vi "OutputShooter.vi"() -> ()   [LabVIEW 2023]
doc: "This VI sends commands to the arm subsystem."
uses:
  f035948c-00ce-4b24-a9d1-78143a22adfc.vi
  GlobalShooter.vi
  GRNF_CTREMotor.vi
  <vilib>/Rock Robotics/WPI/ThirdParty/Phoenix-LabVIEW/Motor Controller/Get/CTRE_Phoenix_MotorController_GetSelectedSensorData.vi
  <vilib>/Rock Robotics/WPI/ThirdParty/Phoenix-LabVIEW/Motor Controller/Get/CTRE_Phoenix_MotorController_GetVoltage.vi
  <vilib>/Rock Robotics/Network Tables/NT Read Number.vi
  <vilib>/Rock Robotics/Network Tables/NT Read Boolean.vi
  <vilib>/Rock Robotics/WPI/ThirdParty/Phoenix-LabVIEW/Motor Controller/Get/CTRE_Phoenix_MotorController_GetGeneralStatus.vi
  GlobalDriverStationData.vi
  GlobalElevator.vi
  GlobalDriverStationCommands.vi
panel:
  in  "Wrist Homing Power":dbl=-0.1 format="%#_13g"
  in  "Shootering?":bool=TRUE
  in  "OUT_Wrist_PID_Mode Override":T1(ring)=enum."Positioning"
  out "Error Chart":dbl(graph)=-0.3784677933673469
  out "Angle Chart":dbl(graph)=-0.3784677933673469
  out "Wrist Error":dbl=-0.3784677933673469
  in  "Wrist output override":bool
  in  "OUT_Shooter_Wrist":dbl
  in  "Shooter Right PID Configuration":T2
  in  "Shooter Left PID Configuration":T2
  in  "Manual Shooter Right Speed Goal (rpm)":dbl min=0.0 max=6000.0 step=100.0
  in  "Manual Shooter Left Speed Goal (rpm)":dbl min=0.0 max=6000.0 step=100.0
  in  "Override Shooter State Controller":bool
  out "Shooter Right":T3(graph)
  out "Shooter Left":T3(graph)
  in  "Plot Shooter":bool
  in  "Wrist Scalar":dbl=0.008
  in  "Wrist Positioning PID Parameters":T2={"Kp"=0.060000000000000005, "Ki"=0.0, "Kd"=0.0, "Kf (don't use)"=0.0, "I-Zone"=10.0} {"Kd" min=0.0; "Ki" min=0.0; "Kp" min=0.0}
  in  "Wrist Acceleration (deg/s^2)":dbl=550.0
  in  "Wrist S-Curve Strength":dbl=4.0
  in  "Wrist Cruise Velocity (deg/s)":dbl=350.0
  in  "Wrist Travelling PID Parameters":T2={"Kp"=0.05, "Ki"=1e-05, "Kd"=0.0, "Kf (don't use)"=0.0, "I-Zone"=10.0} {"Kd" min=0.0; "Ki" min=0.0; "Kp" min=0.0}
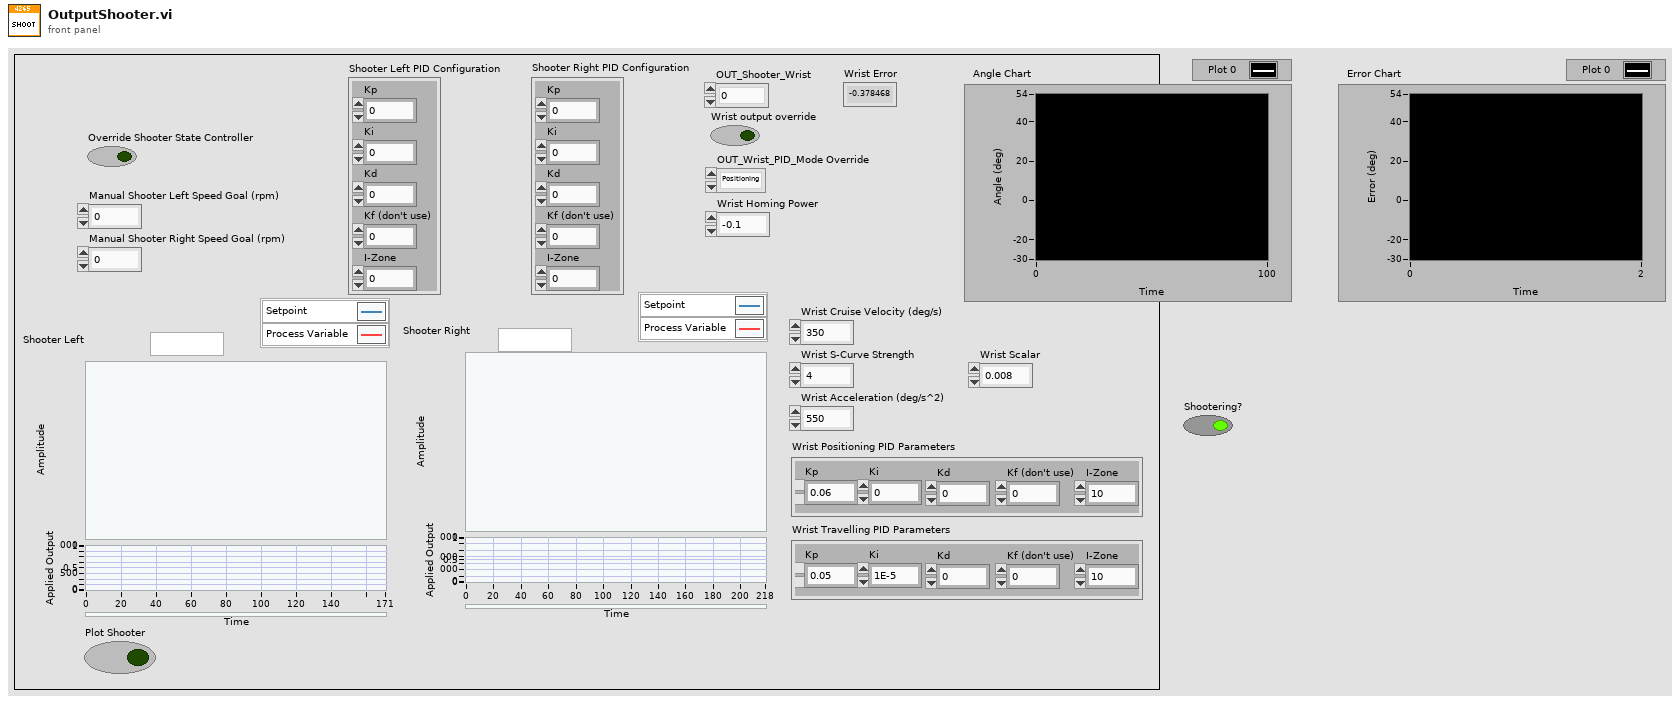
[diagram p1: front panel]
types:
  T1 = enum16{"Safety", "Travelling", "Positioning", "Holding"}
  T2 = cluster{"Kp":dbl, "Ki":dbl, "Kd":dbl, "Kf (don't use)":dbl, "I-Zone":dbl}
  T3 = cluster{"Sensor Velocity":dbl, "Setpoint":dbl, "Applied Output":dbl}
  T4 = typedef "WPI_MotorControlDeviceRef.ctl" = cluster{"DeviceStatus":errorcluster, "Type":T5, "PWM":cluster{"PWM Channel":T6, "DeadBand":T7}, "CAN":cluster{"Device Number":u8, "SetOutput VI Ref":variant, "GetOutput VI Ref":variant, "Enable VI Ref":variant, "Disable VI Ref":variant, "Data":variant}, "Invert":bool, "DIO PWM":cluster{"PWM \"Enable\" Channel":T6, "DIOChannel":T8, "PWM Rate":dbl}}
  T5 = typedef "WPI_MotorControlType.ctl" = enum16{"PWM", "CAN", "DIO PWM"}
  T6 = typedef "FPGA_DIOPWMChannel.ctl" = enum8{"PWM 0", "PWM 1", "PWM 2", "PWM 3", "PWM 4", "PWM 5", "PWM 6", "PWM 7", "PWM 8", "PWM 9", "PWM MXP 0", "PWM MXP 1", "PWM MXP 2", "PWM MXP 3", "PWM MXP 4", "PWM MXP 5", "PWM MXP 6", "PWM MXP 7", "PWM MXP 8", "PWM MXP 9", "Invalid"}
  T7 = typedef "WPI_PWMDeadband.ctl" = cluster{"Name":string, "maxPositivePwm":i32, "minPositivePwm":i32, "centerPwm":i32, "maxNegativePwm":i32, "minNegativePwm":i32, "angularRange":u16}
  T8 = typedef "FPGA_DIOChannel.ctl" = enum8{"DIO 0", "DIO 1", "DIO 2", "DIO 3", "DIO 4", "DIO 5", "DIO 6", "DIO 7", "DIO 8", "DIO 9", "DIO MXP 0", "DIO MXP 1", "DIO MXP 2", "DIO MXP 3", "DIO MXP 4", "DIO MXP 5", "DIO MXP 6", "DIO MXP 7", "DIO MXP 8", "DIO MXP 9", "DIO MXP 10", "DIO MXP 11", "DIO MXP 12", "DIO MXP 13", "DIO MXP 14", "DIO MXP 15", "SPI Port CS1", "SPI Port CS2", "SPI Port CS3", "SPI Port MISO", "SPI Port MOSI", "Invalid"}
  T9 = enum16{"No Changed Output", "New Normal Output", "New Testing Output"}
  T10 = cluster{"Interlocked Output":dbl, dbl, "Percent Output":dbl}
  T11 = typedef "WPI_SolenoidDevRef.ctl" = cluster{"DevStatus":errorcluster, "Pneumatics Control Module":u8, "Forward Solenoid Channel":T12, "Reverse Solenoid Channel":T12}
  T12 = typedef "WPI_SolenoidChannel.ctl" = enum8{"Solenoid 0", "Solenoid 1", "Solenoid 2", "Solenoid 3", "Solenoid 4", "Solenoid 5", "Solenoid 6", "Solenoid 7", "Solenoid 8", "Solenoid 9", "Solenoid 10", "Solenoid 11", "Solenoid 12", "Solenoid 13", "Solenoid 14", "Solenoid 15", "Invalid"}
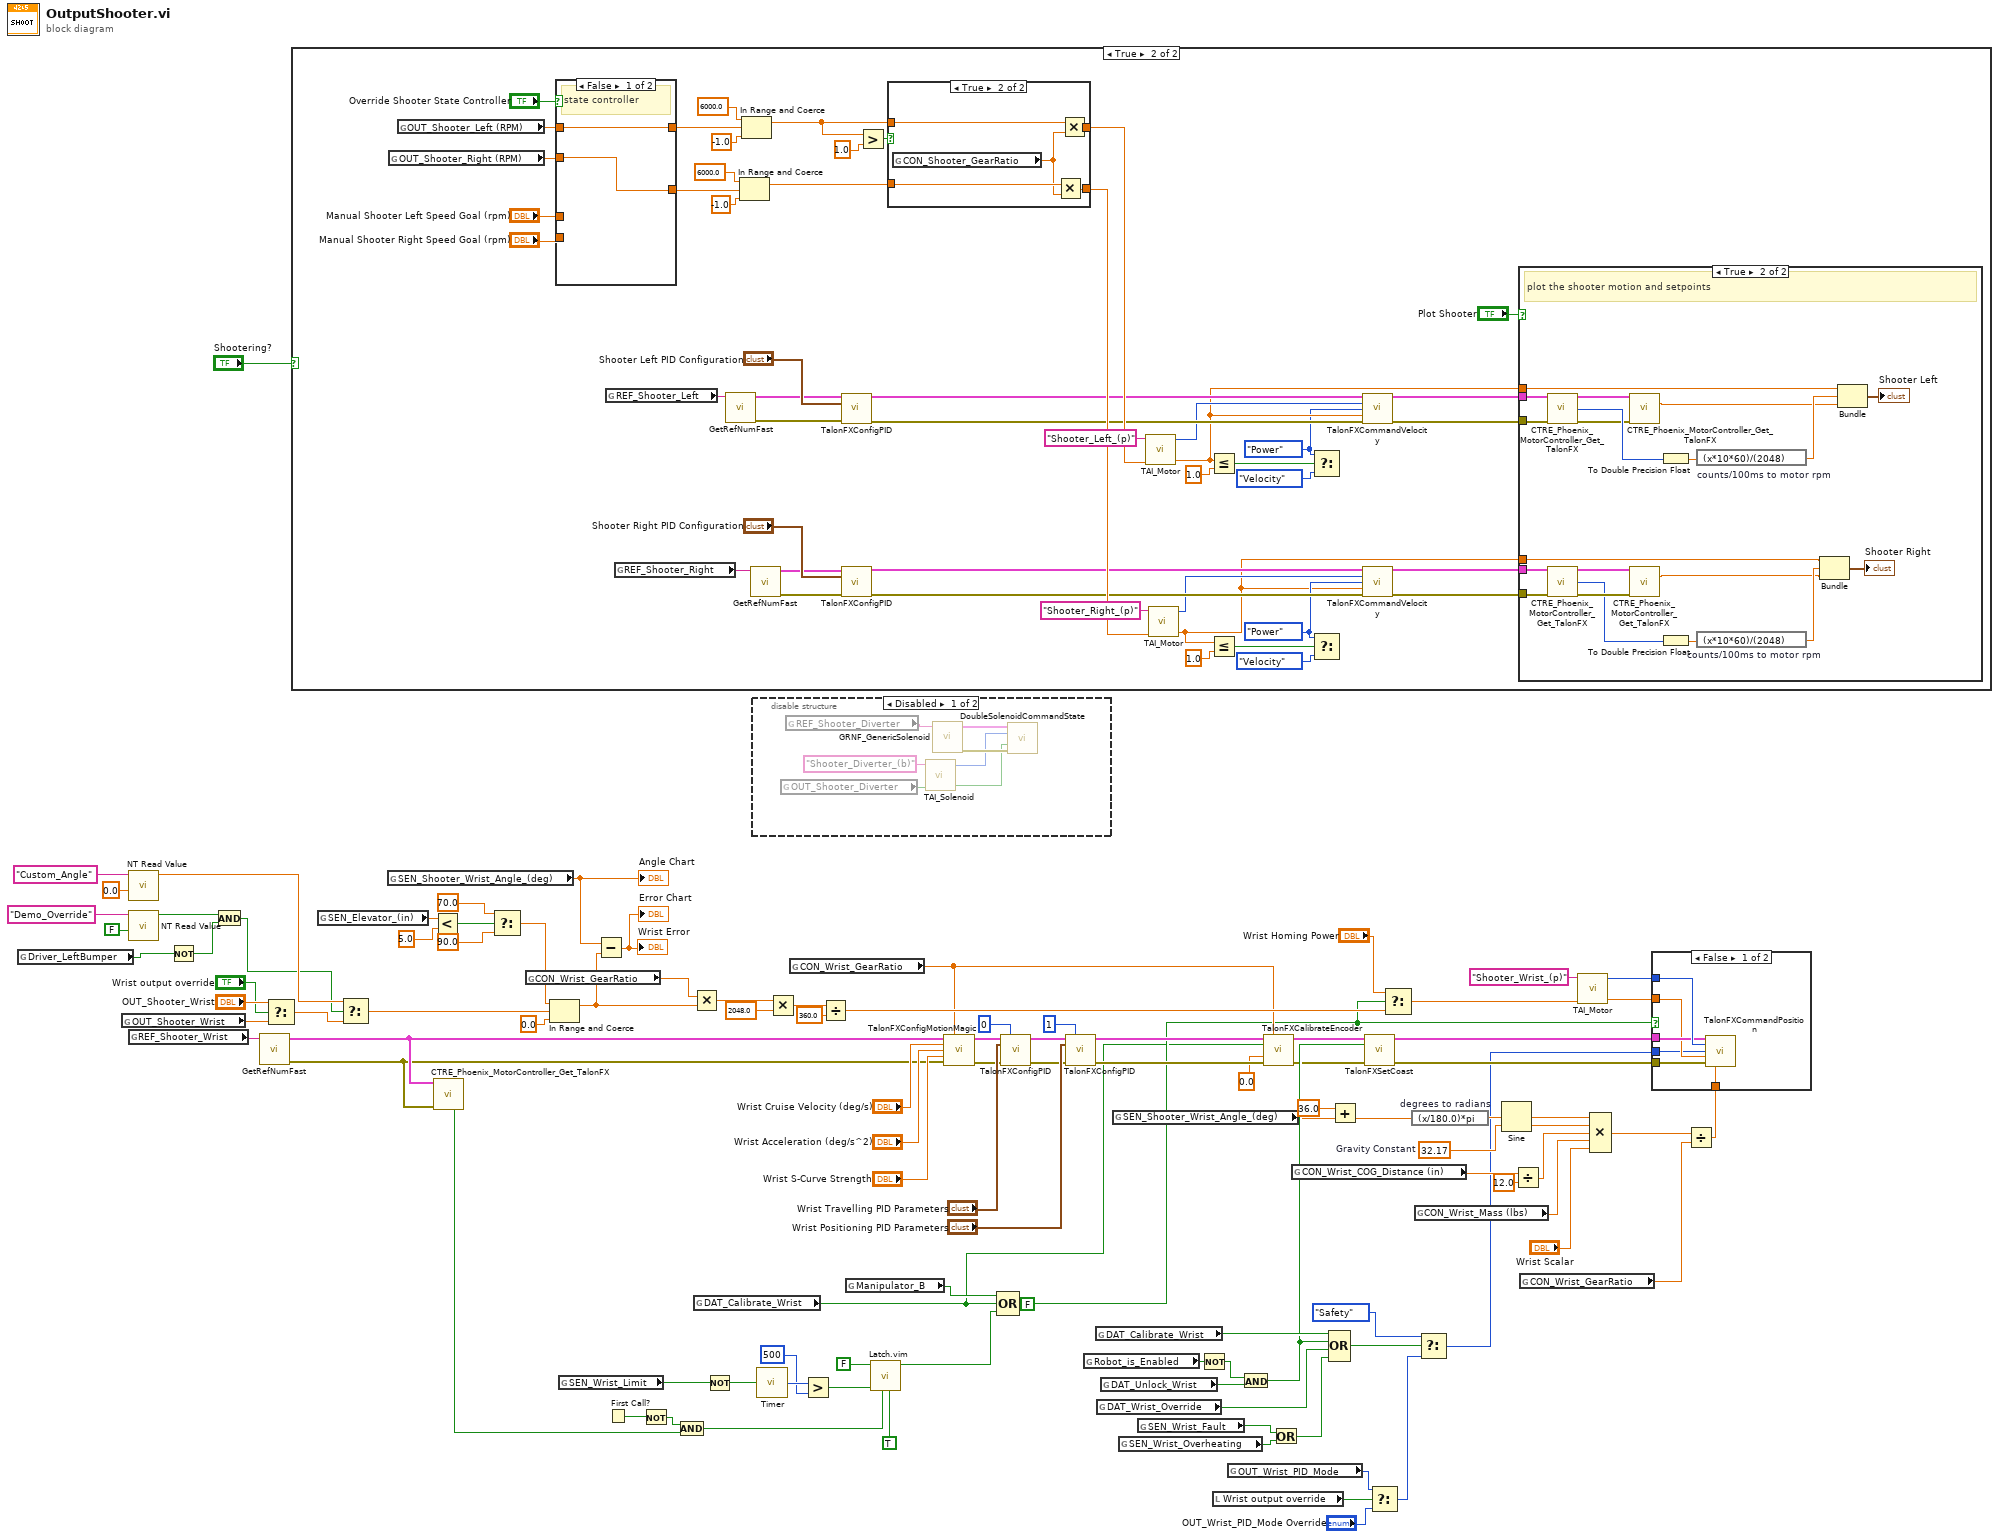
[diagram p0: block diagram]
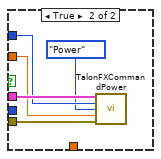
[diagram p2: hidden frame]
diagram:
  w13 = FALSE
  w78 = 32.17  # Gravity Constant
  n1 = global read "GlobalDriverStationCommands.vi" "Driver_LeftBumper"() -> (w3:bool)
  n2 = global read "GlobalShooter.vi" "OUT_Shooter_Wrist"() -> (w65:dbl)
  n3 = call-poly <vilib>:"NT Read Value.vi"("default value"=0.0, "name"="Custom_Angle") -> ("value"=w6:dbl)  [unwired: 7 in, 2 out]
  n4 = call-poly <vilib>:"NT Read Value.vi"("default value"=FALSE, "name"="Demo_Override") -> ("value"=w4:bool)  [unwired: 7 in, 2 out]
  n5 = global read "GlobalShooter.vi" "REF_Shooter_Wrist"() -> (w102:string)
  n6 = Not(x=w3) -> (.not. x?=w2:bool)
  n7 = And(x=w4, y=w2) -> (x .and. y?=w1:bool)
  n8 = call-poly "GetRefNumFast.vi"("RefNum Name"=w102) -> ("Error"=w27:errorcluster, "Device Reference"=w28:T4)  [unwired: 5 in]
  n9 = Select(t="OUT_Shooter_Wrist", s="Wrist output override", f=w65) -> (s? t:f=w11:dbl)
  n10 = case shown="True" "Shootering?" {
    frame False {
    }
    frame True {
      w110 = enum16{"Safety", "Power", "Velocity"}."Power" ("Control Mode")
      w117 = enum16{"Safety", "Power", "Velocity"}."Power" ("Control Mode")
      n11 = global read "GlobalShooter.vi" "OUT_Shooter_Right (RPM)"() -> (w139:dbl)
      n12 = global read "GlobalShooter.vi" "OUT_Shooter_Left (RPM)"() -> (w140:dbl)
      n13 = case shown="False" "Override Shooter State Controller" {
        tunnel: "Manual Shooter Left Speed Goal (rpm)" -> [_ w182]
        tunnel: "Manual Shooter Right Speed Goal (rpm)" -> [_ w181]
        tunnel: w139 -> [w179 _]
        tunnel: w140 -> [w180 _]
        tunnel: [w180 w182] -> w146
        tunnel: [w179 w181] -> w143
        frame False {
          # "state controller"
        }
        frame True {
          # "manual control"
        }
      }
      n14 = global read "GlobalShooter.vi" "REF_Shooter_Left"() -> (w137:string)
      n15 = global read "GlobalShooter.vi" "REF_Shooter_Right"() -> (w138:string)
      n16 = call-poly "GetRefNumFast.vi"("RefNum Name"=w137) -> ("Error"=w124:errorcluster, "Device Reference"=w125:T4)  [unwired: 5 in]
      n17 = In Range and Coerce(upper limit=6000.0, x=w143, lower limit=-1.0) -> (coerced(x)=w129:dbl)  [unwired: 1 out]
      n18 = In Range and Coerce(upper limit=6000.0, x=w146, lower limit=-1.0) -> (coerced(x)=w105:dbl)  [unwired: 1 out]
      n19 = call-poly "GetRefNumFast.vi"("RefNum Name"=w138) -> ("Error"=w114:errorcluster, "Device Reference"=w115:T4)  [unwired: 5 in]
      n20 = call "TalonFXConfigPID.vi"("Device Reference (in)"=w125, "PID Parameters"="Shooter Left PID Configuration", "Error (in)"=w124) -> ("Device Reference (out)"=w123:T4, "Error (out)"=w122:errorcluster)  [unwired: 11 in]
      n21 = call "TalonFXConfigPID.vi"("Device Reference (in)"=w115, "PID Parameters"="Shooter Right PID Configuration", "Error (in)"=w114) -> ("Device Reference (out)"=w113:T4, "Error (out)"=w112:errorcluster)  [unwired: 11 in]
      n22 = Greater?(x=w105, y=1.0) -> (0:w104:bool)
      n23 = case shown="True" w104 {
        tunnel: w105 -> [w153 w158]
        tunnel: [w153 w157] -> w130
        tunnel: w129 -> [w152 w156]
        tunnel: [w152 w155] -> w128
        frame False {
        }
        frame True {
          n24 = global read "GlobalShooter.vi" "CON_Shooter_GearRatio"() -> (w154:dbl)
          n25 = Multiply(x=w156, y=w154) -> (x*y=w155:dbl)
          n26 = Multiply(x=w158, y=w154) -> (x*y=w157:dbl)
        }
      }
      n27 = call "TAI_Motor.vi"("Normal Output"=w130, "Actuator Name"="Shooter_Left_(p)" ("Actuator_Name")) -> ("Interlocked Output"=w120:dbl, "Testing Mode"=w121:T9)  [unwired: 3 in]
      n28 = call "TAI_Motor.vi"("Normal Output"=w128, "Actuator Name"="Shooter_Right_(p)" ("Actuator_Name")) -> ("Interlocked Output"=w109:dbl, "Testing Mode"=w111:T9)  [unwired: 3 in]
      n29 = Less Or Equal?(x=w120, y=1.0) -> (x <= y?=w135:bool)
      n30 = Less Or Equal?(x=w109, y=1.0) -> (x <= y?=w132:bool)
      n31 = Select(t=w117, s=w135, f=enum16{"Safety", "Power", "Velocity"}."Velocity" ("Control Mode")) -> ()  [unwired: 1 out]
      n32 = Select(t=w110, s=w132, f=enum16{"Safety", "Power", "Velocity"}."Velocity" ("Control Mode")) -> ()  [unwired: 1 out]
      n33 = call "TalonFXCommandVelocity.vi"("Device Reference (in)"=w123, "Output Mode"=w121, "Control Mode"=w117, "Velocity, Power, or Testing Power"=w120, "Error (in)"=w122) -> ("Device Reference (out)"=w119:T4, "Error (out)"=w118:errorcluster)  [unwired: 9 in]
      n34 = call "TalonFXCommandVelocity.vi"("Device Reference (in)"=w113, "Output Mode"=w111, "Control Mode"=w110, "Velocity, Power, or Testing Power"=w109, "Error (in)"=w112) -> ("Device Reference (out)"=w107:T4, "Error (out)"=w108:errorcluster)  [unwired: 9 in]
      n35 = case shown="True" "Plot Shooter" {
        tunnel: w120 -> [_ w178]
        tunnel: w119 -> [_ w169]
        tunnel: w107 -> [_ w162]
        tunnel: w109 -> [_ w172]
        tunnel: w108 -> [_ w161]
        tunnel: w118 -> [_ w168]
        frame False {
          # "disable plotting and expensive sensor polling"
        }
        frame True {
          # "plot the shooter motion and setpoints"
          n36 = call-poly <vilib>:"CTRE_Phoenix_MotorController_Get_TalonFX.vi"("PhoenixMotorControlDevRef"=w169, "error in"=w168) -> ("PhoenixMotorControlDevRef"=w166:T4, "Velocity (Raw Sensor Units per 100 ms)"=w170:i32, "error out"=w165:errorcluster)  [unwired: 10 in, 1 out]
          n37 = call-poly <vilib>:"CTRE_Phoenix_MotorController_Get_TalonFX.vi"("PhoenixMotorControlDevRef"=w162, "error in"=w161) -> ("PhoenixMotorControlDevRef"=w163:T4, "Velocity (Raw Sensor Units per 100 ms)"=w159:i32, "error out"=w164:errorcluster)  [unwired: 10 in, 1 out]
          n38 = call-poly <vilib>:"CTRE_Phoenix_MotorController_Get_TalonFX.vi"("PhoenixMotorControlDevRef"=w166, "error in"=w165) -> ("Percent Output"=w167:dbl)  [unwired: 9 in, 4 out]
          n39 = call-poly <vilib>:"CTRE_Phoenix_MotorController_Get_TalonFX.vi"("PhoenixMotorControlDevRef"=w163, "error in"=w164) -> ("Percent Output"=w160:dbl)  [unwired: 9 in, 4 out]
          n40 = To Double Precision Float(number=w170) -> (double precision float=w177:dbl)
          n41 = To Double Precision Float(number=w159) -> (double precision float=w173:dbl)
          n42 = expression code="(x*10*60)/(2048)" "counts/100ms to motor rpm"(w177) -> (w176:dbl)
          n43 = expression code="(x*10*60)/(2048)" "counts/100ms to motor rpm"(w173) -> (w171:dbl)
          n44 = Bundle("Interlocked Output"=w172, w171, "Percent Output"=w160) -> (→"Shooter Right":T10)  [unwired: 1 in]
          n45 = Bundle("Interlocked Output"=w178, w176, "Percent Output"=w167) -> (→"Shooter Left":T10)  [unwired: 1 in]
        }
      }
    }
  }
  n46 = global read "GlobalElevator.vi" "SEN_Elevator_(in)"() -> (w51:dbl)
  n47 = Select(t=w6, s=w1, f=w11) -> (s? t:f=w5:dbl)
  n48 = global read "GlobalShooter.vi" "SEN_Shooter_Wrist_Angle_(deg)"() -> (w67:dbl)
  "Angle Chart" <- w67
  n49 = Less?(x=w51, y=5.0) -> (x < y?=w49:bool)
  n50 = call-poly <vilib>:"CTRE_Phoenix_MotorController_Get_TalonFX.vi"("PhoenixMotorControlDevRef"=w28, "error in"=w27) -> ("Has Reset Occurred?"=w24:bool)  [unwired: 8 in, 5 out]
  n51 = Select(t=70.0, s=w49, f=90.0) -> (s? t:f=w44:dbl)
  n52 = global read "GlobalShooter.vi" "CON_Wrist_GearRatio"() -> (w37:dbl)
  n53 = In Range and Coerce(upper limit=w44, x=w5, lower limit=0.0) -> (coerced(x)=w53:dbl)  [unwired: 1 out]
  n54 = global read "GlobalShooter.vi" "SEN_Wrist_Limit"() -> (w19:bool)
  n55 = Subtract(x=w67, y=w53) -> (x-y=→"Wrist Error" →"Error Chart":dbl)
  n56 = First Call?() -> (First Call?: T/F=w26:bool)
  n57 = Not(x=w26) -> (.not. x?=w25:bool)
  n58 = And(x=w25, y=w24) -> (x .and. y?=w23:bool)
  n59 = Multiply(x=w37, y=w53) -> (x*y=w60:dbl)
  n60 = global read "GlobalShooter.vi" "DAT_Calibrate_Wrist"() -> (w12:bool)
  n61 = Not(x=w19) -> (.not. x?=w34:bool)
  n62 = disable-structure shown="Disabled" {
    frame Disabled {
      n63 = global read "GlobalShooter.vi" "OUT_Shooter_Diverter"() -> (w183:bool)
      n64 = global read "GlobalShooter.vi" "REF_Shooter_Diverter"() -> (w184:string)
      n65 = call "TAI_Solenoid.vi"("Normal Output"=w183, "Actuator Name"="Shooter_Diverter_(b)") -> ("Interlocked Output"=w185:bool, "Output Mode"=w186:T9)  [unwired: 3 in]
      n66 = call "GRNF_GenericSolenoid.vi"("RefNum Name"=w184) -> ("Error"=w187:errorcluster, "Device Reference"=w188:T11)  [unwired: 5 in]
      n67 = call "DoubleSolenoidCommandState.vi"("Device Reference (in)"=w188, "Output Mode"=w186, "State [True, False]"=w185, "Error (in)"=w187) -> ()  [unwired: 12 in]
    }
    frame Enabled {
    }
  }
  n68 = call "Timer.vi"("Reset Timer"=w34) -> ("Time (ms)"=w33:u32)
  n69 = Multiply(x=w60, y=2048.0) -> (x*y=w57:dbl)
  n70 = global read "GlobalShooter.vi" "CON_Wrist_GearRatio"() -> (w18:dbl)
  n71 = Greater?(x=w33, y=u32 500) -> (0:w31:bool)
  n72 = Divide(x=w57, y=360.0) -> (x/y=w22:dbl)
  n73 = global read "GlobalDriverStationCommands.vi" "Manipulator_B"() -> (w29:bool)
  n74 = call "Latch.vim"("Default Value"=TRUE ("Reset"), "Reset"=w23, "Latch Signal"=w31, "Latch Value"=FALSE ("Reset")) -> ("Latched"=w30:bool)  [unwired: 7 in]
  n75 = call "TalonFXConfigMotionMagic.vi"("Device Reference (in)"=w28, "Gear Ratio"=w18, "Cruise Velocity (deg/s)"="Wrist Cruise Velocity (deg/s)", "Acceleration (deg/s^2)"="Wrist Acceleration (deg/s^2)", "S-Curve Strength"="Wrist S-Curve Strength", "Error (in)"=w27) -> ("Device Reference (out)"=w97:T4, "Error (out)"=w98:errorcluster)  [unwired: 8 in]
  n76 = Compound Arithmetic op=OR(w29, w12, w30) -> ()  [unwired: 1 out]
  n77 = call "TalonFXConfigPID.vi"("Device Reference (in)"=w97, "PID Slot"=0, "PID Parameters"="Wrist Travelling PID Parameters", "Error (in)"=w98) -> ("Device Reference (out)"=w91:T4, "Error (out)"=w90:errorcluster)  [unwired: 10 in]
  n78 = call "TalonFXConfigPID.vi"("Device Reference (in)"=w91, "PID Slot"=1, "PID Parameters"="Wrist Positioning PID Parameters", "Error (in)"=w90) -> ("Device Reference (out)"=w41:T4, "Error (out)"=w40:errorcluster)  [unwired: 10 in]
  n79 = global read "GlobalDriverStationData.vi" "Robot_is_Enabled"() -> (w86:bool)
  n80 = global read "GlobalShooter.vi" "DAT_Calibrate_Wrist"() -> (w89:bool)
  n81 = global read "GlobalShooter.vi" "DAT_Wrist_Override"() -> (w88:bool)
  n82 = global read "GlobalShooter.vi" "DAT_Unlock_Wrist"() -> (w87:bool)
  n83 = global read "GlobalShooter.vi" "SEN_Shooter_Wrist_Angle_(deg)"() -> (w61:dbl)
  n84 = global read "GlobalShooter.vi" "SEN_Wrist_Overheating"() -> (w83:bool)
  n85 = global read "GlobalShooter.vi" "SEN_Wrist_Fault"() -> (w84:bool)
  n86 = Not(x=w86) -> (.not. x?=w85:bool)
  n87 = local read "Wrist output override"() -> (w17:bool)
  n88 = global read "GlobalShooter.vi" "OUT_Wrist_PID_Mode"() -> (w16:T1)
  n89 = And(x=w85, y=w87) -> (x .and. y?=w64:bool)
  n90 = call "TalonFXCalibrateEncoder.vi"("Device Reference (in)"=w41, "Gear Ratio"=w18, "Calibration Trigger"=w12, "Calibration Angle (deg)"=0.0, "Error (in)"=w40) -> ("Device Reference (out)"=w42:T4, "Error (out)"=w39:errorcluster)  [unwired: 8 in, 1 out]
  n91 = Or(x=w84, y=w83) -> (x .or. y?=w82:bool)
  n92 = global read "GlobalShooter.vi" "CON_Wrist_COG_Distance (in)"() -> (w70:dbl)
  n93 = Compound Arithmetic op=OR(w89, w64, w88, w82) -> (w81:bool)
  n94 = Add(x=36.0, y=w61) -> (x+y=w55:dbl)
  n95 = call "TalonFXSetCoast.vi"("Device Reference (in)"=w42, "Set Coast Mode"=w64, "Error (in)"=w39) -> ("Device Reference (out)"=w79:T4, "Error (out)"=w80:errorcluster)  [unwired: 11 in]
  n96 = Select(t=w16, s=w17, f="OUT_Wrist_PID_Mode Override") -> (s? t:f=w14:T1)
  n97 = Select(t="Wrist Homing Power", s=w13, f=w22) -> (s? t:f=w20:dbl)
  n98 = expression code="(x/180.0)*pi" "degrees to radians"(w55) -> (w62:dbl)
  n99 = global read "GlobalShooter.vi" "CON_Wrist_Mass (lbs)"() -> (w77:dbl)
  n100 = Select(t=T1."Safety" ("OUT_Wrist_PID_Mode"), s=w81, f=w14) -> (s? t:f=w45:T1)
  n101 = Sine(x=w62) -> (sin(x)=w63:dbl)
  n102 = Divide(x=w70, y=12.0) -> (x/y=w75:dbl)
  n103 = global read "GlobalShooter.vi" "CON_Wrist_GearRatio"() -> (w73:dbl)
  n104 = call "TAI_Motor.vi"("Normal Output"=w20, "Actuator Name"="Shooter_Wrist_(p)") -> ("Interlocked Output"=w58:dbl, "Testing Mode"=w100:T9)  [unwired: 3 in]
  n105 = Compound Arithmetic op=MULTIPLY(w63, w78, w75, w77, "Wrist Scalar") -> (w74:dbl)
  n106 = Divide(x=w74, y=w73) -> (x/y=w72:dbl)
  n107 = case shown="False" w13 {
    tunnel: w100 -> [w195 w197]
    tunnel: w80 -> [w194 w199]
    tunnel: w79 -> [w193 w200]
    tunnel: w72 -> [w192 _]
    tunnel: w58 -> [w191 w198]
    tunnel: w45 -> [w190 _]
    frame False {
      n108 = call "TalonFXCommandPosition.vi"("Device Reference (in)"=w193, "Output Mode"=w195, "Control Mode"=w190, "Position (counts) or Testing Power"=w191, "Error (in)"=w194, "Feed Forward Power [-1, 1]"=w192) -> ()  [unwired: 10 in]
    }
    frame True {
      n109 = call "TalonFXCommandPower.vi"("Device Reference (in)"=w200, "Output Mode"=w197, "Control Mode"=enum16{"Safety", "Power"}."Power", "Power or Testing Power"=w198, "Error (in)"=w199) -> ()  [unwired: 11 in]
    }
  }
